vi "Save Data.vi"(7 "时间标识":timestamp, 9 "数据标记":string, 10 "测试人员":string, 11 "扫描数据":dbl[][](array[numeric])) -> ()   [LabVIEW 2019]
uses:
  <vilib>/Utility/file.llb/Write Delimited Spreadsheet (DBL).vi
  <vilib>/ErrorRing/Error Ring.xnode
panel:
  # "时间\n\n电压\n\n电流"
  # "文件名：日期-时间-数据标记"
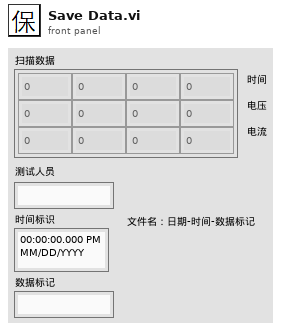
[diagram p1: front panel]
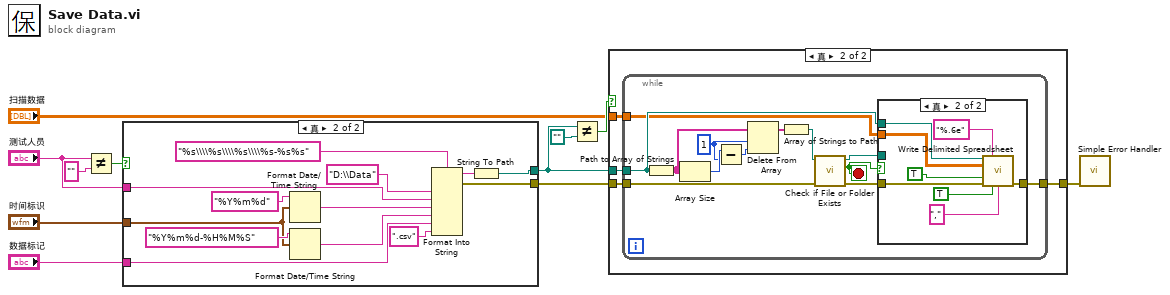
[diagram p0: block diagram]
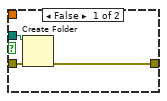
[diagram p3: hidden frame]
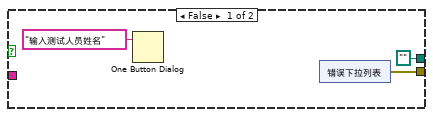
[diagram p4: hidden frame]
diagram:
  n1 = Not Equal?(x="测试人员", y="") -> (x != y?=w9:bool)
  n2 = case shown="真" w9 {
    tunnel: [path "" w25] -> w8
    tunnel: "测试人员" -> [_ w24]
    tunnel: "数据标记" -> [_ w20]
    tunnel: "时间标识" -> [_ w18]
    tunnel: [w12 w16] -> w2
    frame False {
      n3 = One Button Dialog(message="输入测试人员姓名" ("消息")) -> ()  [unwired: 1 in, 1 out]
      n4 = xnode "错误下拉列表"() -> ("错误输出"=w12:errorcluster)
    }
    frame True {
      n5 = Format Date/Time String(time format string (%c)="%Y%m%d" ("时间格式字符串(%c)"), seconds (now)=w18) -> (date/time string=w22:string)  [unwired: 1 in]
      n6 = Format Date/Time String(time format string (%c)="%Y%m%d-%H%M%S" ("时间格式字符串(%c)"), seconds (now)=w18) -> (date/time string=w21:string)  [unwired: 1 in]
      n7 = Format Into String(format string="%s\\\\%s\\\\%s\\\\%s-%s%s" ("格式字符串"), "D:\\Data", w24, w22, w21, w20, ".csv") -> (resulting string=w28:string, error out=w16:errorcluster)  [unwired: 2 in]
      n8 = String To Path(string=w28) -> (path=w25:path)
    }
  }
  n9 = Not Equal?(x=w8, y=path "") -> (x != y?=w6:bool)
  n10 = case shown="真" w6 {
    tunnel: w8 -> [_ w33]
    tunnel: "扫描数据" -> [_ w32]
    tunnel: [w29 w31] -> w1
    tunnel: w2 -> [w29 w30]
    frame False {
    }
    frame True {
      n11 = while {
        tunnel: w33 -> [w46]
        tunnel: w32 -> [w36]
        tunnel: [w35] -> w31
        tunnel: w30 -> [w34]
        stop <- w39 stop-if-true
        w43 = 1 ("长度")
        n12 = Path to Array of Strings(0:w46) -> (2:w45:string[])  [unwired: 1 out]
        n13 = Array Size(array=w45) -> (size(s)=w44:i32)
        n14 = Subtract(x=w44, y=w43) -> (x-y=w42:i32)
        n15 = Delete From Array(array=w45, length=w43, index=w42) -> (array with subset deleted=w41:string[])  [unwired: 1 out]
        n16 = Array of Strings to Path(0:w41) -> (2:w40:path)  [unwired: 1 in]
        n17 = call <vilib>:"Check if File or Folder Exists.vi"("error in (no error)"=w34, "path"=w40) -> ("error out"=w37:errorcluster, "file or folder exists?"=w39:bool, "dup path"=w38:path)  [unwired: 7 in]
        n18 = case shown="真" w39 {
          tunnel: w46 -> [_ w53]
          tunnel: w38 -> [w49 _]
          tunnel: w37 -> [w48 w51]
          tunnel: w36 -> [_ w52]
          tunnel: [w47 w50] -> w35
          frame False {
            n19 = Create Folder(path (use dialog)=w49, error in=w48) -> (error out=w47:errorcluster)  [unwired: 1 in, 2 out]
          }
          frame True {
            n20 = call-poly <vilib>:"Write Delimited Spreadsheet.vi"("file path (dialog if empty)"=w53, "format (%.3f)"="%.6e", "2D data"=w52, "append to file? (new file:F)"=TRUE, "error in (no error)"=w51, "transpose? (no:F)"=TRUE, "delimiter (\\t)"="," ("delimiter (\\t)")) -> ("error out"=w50:errorcluster)  [unwired: 7 in, 1 out]
          }
        }
      }
    }
  }
  n21 = call <vilib>:"Simple Error Handler.vi"("error in (no error)"=w1) -> ()  [unwired: 4 in, 5 out]
